vi "OAT Get Baseline Property.vi"(10 "baseline":cluster{"r0":dbl, "dr":dbl, "Y":dbl[]} {"Y" format="%.2f"; "dr" format="%.2f"; "r0" format="%.2f"}) -> (1 "samples":i32, 2 "samples/rev":i32)   [LabVIEW 2017]
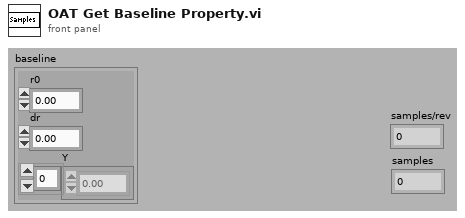
[diagram p1: front panel]
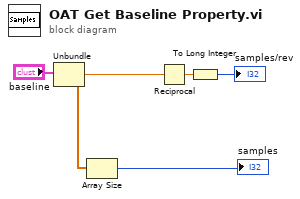
[diagram p0: block diagram]
diagram:
  n1 = Unbundle("baseline") -> ("dr"=w4:dbl, "Y"=w6:dbl[])  [unwired: 1 out]
  n2 = Array Size(array=w6) -> (size(s)=→"samples":i32)
  n3 = Reciprocal(x=w4) -> (1/x=w3:dbl)
  n4 = To Long Integer(number=w3) -> (32bit integer=→"samples/rev":i32)
